vi "GetNotesHTML.vi"(11 "text":string) -> (3 "Array":string[](array[string]))   [LabVIEW 2018, in "DS_Lib.lvlib" / "SRNotesParser.lvlib"]
uses:
  SRNotesParser.lvlib
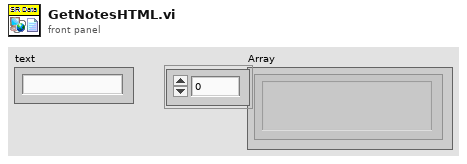
[diagram p1: front panel]
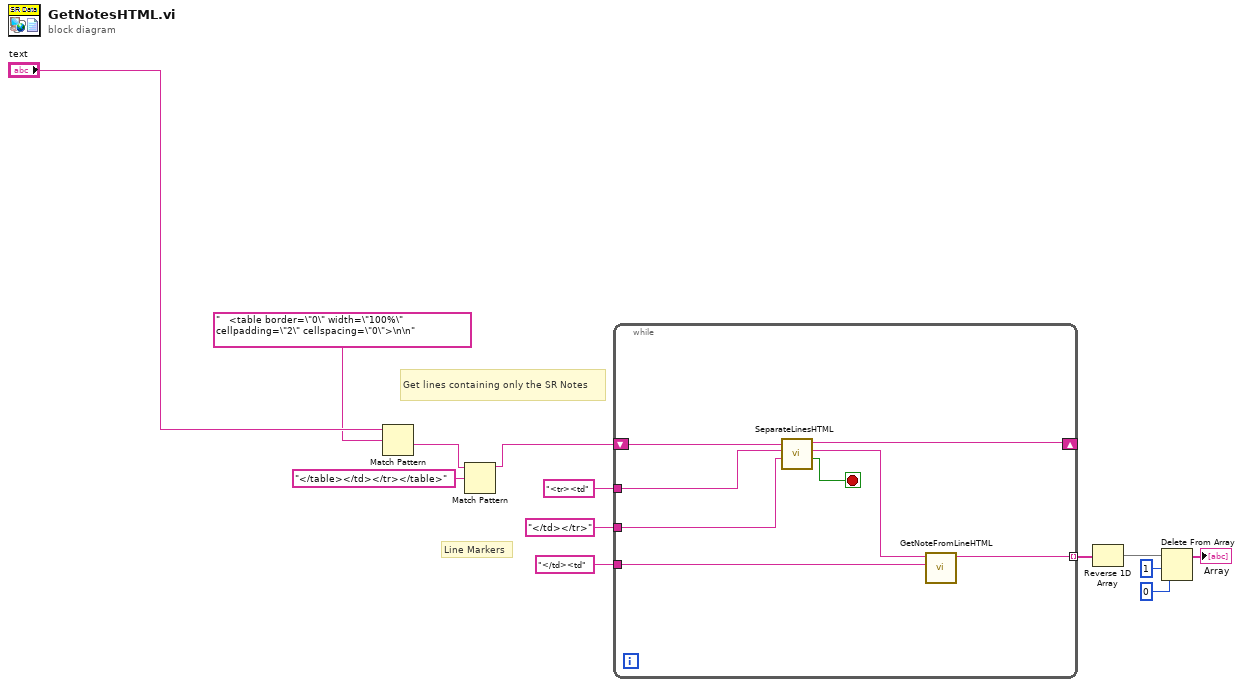
[diagram p0: block diagram]
diagram:
  # "Line Markers"
  # "Get lines containing only the SR Notes"
  n1 = Match Pattern(string="text", regular expression="   <table border=\"0\" width=\"100%\" cellpadding=\"2\" cellspacing=\"0\">\n\n") -> (after substring=w7:string)  [unwired: 1 in, 3 out]
  n2 = Match Pattern(string=w7, regular expression="</table></td></tr></table>") -> (before substring=w9:string)  [unwired: 1 in, 3 out]
  n3 = while {
    shift-right: [w18] -> _
    shift-left: w9 -> [w21]
    tunnel: [w20] -> w3 mode=indexing
    tunnel: "</td><td" ("regular expression") -> [w19]
    tunnel: "</td></tr>" ("regular expression") -> [w15]
    tunnel: "<tr><td" ("regular expression") -> [w14]
    stop <- w16 stop-if-true
    n4 = call "SeparateLinesHTML.vi"("Line end marker"=w15, "Line start marker"=w14, "Input String"=w21) -> ("End of Sting ?"=w16:bool, "Line Out"=w17:string, "Remaining String"=w18:string)  [unwired: 6 in]
    n5 = call "GetNoteFromLineHTML.vi"("Regular Expression (Separator)"=w19, "HTML Line"=w17) -> ("String out"=w20:string)  [unwired: 9 in]
  }
  n6 = Reverse 1D Array(array=w3) -> (reversed array=w2:string[])
  n7 = Delete From Array(array=w2, length=1, index=0) -> (array with subset deleted=→"Array":string[])  [unwired: 1 out]
